vi "Path Ubication.vi"() -> (2 "path string":string, 3 "path":path)   [LabVIEW 2025, in "Control de MaP.lvlib"]
uses:
  Control de MaP.lvlib
  <vilib>/Utility/sysdir.llb/System Directory Type.ctl
panel:
  out "error out":errorcluster
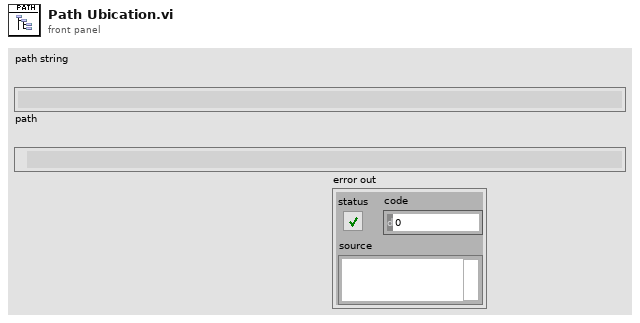
[diagram p1: front panel]
types:
  T1 = typedef "System Directory Type.ctl" = i32
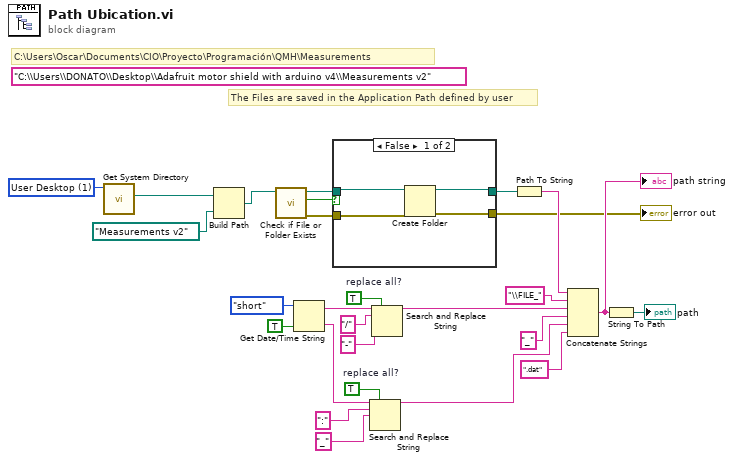
[diagram p0: block diagram]
diagram:
  w7 = TRUE  # replace all?
  w11 = TRUE  # replace all?
  w20 = T1 1 items=["User Home"=0, "User Desktop"=1, "User Documents"=2, "User Application Data"=3, "User Preferences"=4, "User Temporary"=5, "Public Documents"=6, "Public Application Data"=7, "Public Preferences"=8, "Public Cache"=13, "System Core Libraries"=9, "System Installed Libraries"=10, "Application Files"=11, "Boot Volume Root"=12] ("system directory type")
  (unwired) "C:\\Users\\DONATO\\Desktop\\Adafruit motor shield with arduino v4\\Measurements v2"
  # "C:\\Users\\Oscar\\Documents\\CIO\\Proyecto\\Programación\\QMH\\Measurements"
  # "The Files are saved in the Application Path defined by user"
  n1 = call <vilib>:"Get System Directory.vi"("system directory type"=w20) -> ("system directory"=w19:path)  [unwired: 10 in]
  n2 = Build Path(base path=w19, name or relative path=path "Measurements v2") -> (appended path=w6:path)
  n3 = call <vilib>:"Check if File or Folder Exists.vi"("path"=w6) -> ("error out"=w2:errorcluster, "file or folder exists?"=w5:bool, "dup path"=w4:path)  [unwired: 8 in]
  n4 = Get Date/Time String(date format (0)=enum16{"short", "long", "abbreviated"}."short", want seconds? (F)=TRUE) -> (date string=w9:string, time string=w16:string)  [unwired: 1 in]
  n5 = case shown="False" w5 {
    tunnel: w4 -> [w31 w33]
    tunnel: [w30 w33] -> w3
    tunnel: w2 -> [w29 w32]
    tunnel: [w28 w32] -> w1
    frame False {
      n6 = Create Folder(path (use dialog)=w31, error in=w29) -> (created path=w30:path, error out=w28:errorcluster)  [unwired: 1 in, 1 out]
    }
    frame True {
    }
  }
  "error out" <- w1
  n7 = Search and Replace String(replace all?=w11, input string=w16, search string=":", replace string="_" ("replace string (\"\")")) -> (result string=w10:string)  [unwired: 4 in, 3 out]
  n8 = Search and Replace String(replace all?=w7, input string=w9, search string="/", replace string="-" ("replace string (\"\")")) -> (result string=w8:string)  [unwired: 4 in, 3 out]
  n9 = Path To String(path=w3) -> (string=w17:string)
  n10 = Concatenate Strings(w17, "\\FILE_" ("string"), w8, "_" ("string"), w10, ".dat" ("string")) -> (w27:string)
  "path string" <- w27
  n11 = String To Path(string=w27) -> (path=→"path":path)
